vi "Get System Experts.vi"(8 "error in (no error)":errorcluster, 11 "Session in":refnum<k21>="localhost") -> (0 "error out":errorcluster, 2 "Supported Experts":T1[](array[typedef]), 3 "Session out":refnum<k21>)   [LabVIEW 2012, in "nisyscfg.lvlib"]
doc: "Returns the experts available on the system."
uses:
  <vilib>/nisyscfg/nisyscfg.lvlib
  <vilib>/nisyscfg/Expert Info.ctl
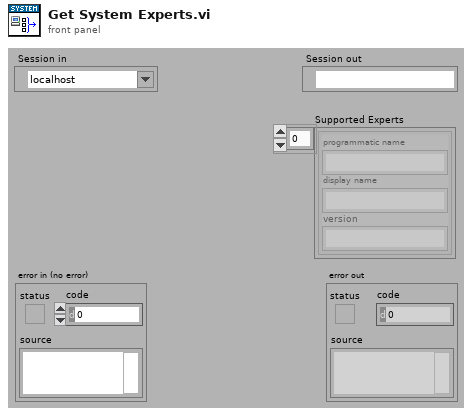
[diagram p1: front panel]
types:
  T1 = typedef "nisyscfg.lvlib/Expert Info.ctl" = cluster{"programmatic name":string, "display name":string, "version":string}
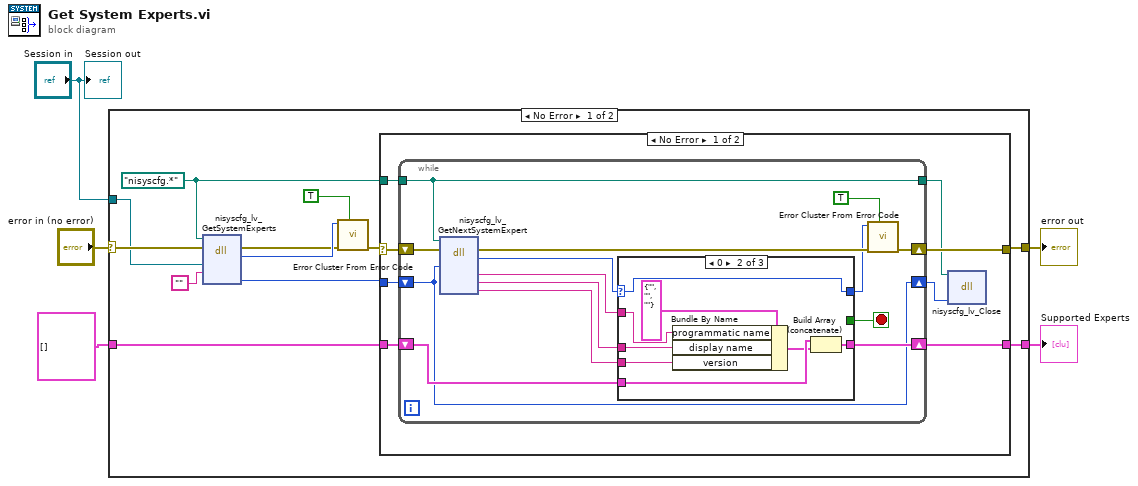
[diagram p0: block diagram]
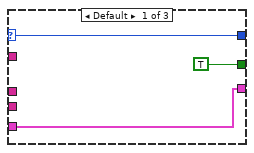
[diagram p2: hidden frame]
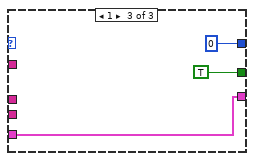
[diagram p3: hidden frame]
diagram:
  n1 = case shown="No Error" "error in (no error)" {
    selector: "error in (no error)" -> [w9 w56]
    tunnel: T1[] [] -> [w14 w57]
    tunnel: [w13 w57] -> w4
    tunnel: [w12 w56] -> w3
    tunnel: "Session in" -> [w8 _]
    frame No Error {
      w7 = path "nisyscfg.*" ("path in")
      n2 = dll-call lib="nisyscfg.*" fn="nisyscfg_lv_GetSystemExperts" label="GetSystemExperts"(path in=w7, error in=w9, "framework"=w8, "experts"="") -> (error out=w16:errorcluster, "status"=w17:i32, "expertsEnum"=w15:u64)  [unwired: 1 in, 4 out]
      n3 = call <vilib>:"Error Cluster From Error Code.vi"("show call chain? (False)"=TRUE, "error in (no error)"=w16, "error code (0)"=w17) -> ("error out"=w11:errorcluster)  [unwired: 6 out]
      n4 = case shown="No Error" w11 {
        selector: w11 -> [w21 w55]
        tunnel: w15 -> [w25 _]
        tunnel: w14 -> [w24 w54]
        tunnel: [w23 w54] -> w13
        tunnel: [w22 w55] -> w12
        tunnel: w7 -> [w19 _]
        frame No Error {
          n5 = while {
            shift-right: [w34] -> w22
            shift-left: w21 -> [w38]
            shift-right: [w32] -> w23
            shift-left: w24 -> [w33]
            shift-right: [w28] -> w20
            shift-left: w25 -> [w28]
            tunnel: w19 -> [w27]
            tunnel: [w27] -> w18
            stop <- w35 stop-if-true
            n6 = dll-call lib="nisyscfg.*" fn="nisyscfg_lv_GetNextSystemExpert" label="GetNextSystemExpert"(path in=w27, error in=w38, "expertsEnum"=w28) -> (error out=w39:errorcluster, "status"=w37:i32, "programmaticName"=w31:string, "displayName"=w30:string, "version"=w29:string)  [unwired: 1 in, 5 out]
            n7 = case shown="0" w37 {
              selector: w37 -> [w42 w50 _]
              tunnel: [w42 w50 0 ("return type")] -> w36
              tunnel: [TRUE _ TRUE] -> w35
              tunnel: w33 -> [w40 w46 w51]
              tunnel: [w40 w44 w51] -> w32
              tunnel: w31 -> [_ w49 _]
              tunnel: w30 -> [_ w48 _]
              tunnel: w29 -> [_ w47 _]
              frame Default {
              }
              frame 0 {
                n8 = Bundle By Name(cluster=T1 {"programmatic name"="", "display name"="", "version"=""} ("expert"), "programmatic name"=w49, "display name"=w48, "version"=w47) -> (w45:T1)
                n9 = Build Array (concatenate)(w46, w45) -> (w44:T1[])
              }
              frame 1 {
              }
            }
            n10 = call <vilib>:"Error Cluster From Error Code.vi"("show call chain? (False)"=TRUE, "error in (no error)"=w39, "error code (0)"=w36) -> ("error out"=w34:errorcluster)  [unwired: 6 out]
          }
          n11 = dll-call lib="nisyscfg.*" fn="nisyscfg_lv_Close" label="Close"(path in=w18, "expertsEnum"=w20) -> ()  [unwired: 3 in, 3 out]
        }
        frame Error {
        }
      }
    }
    frame Error {
    }
  }
  "error out" <- w3
  "Supported Experts" <- w4
  "Session out" <- "Session in"
